vi "Sweep Control Cartesian.vi"() -> ()   [LabVIEW 2019, in "SMO.SweepControl.lvclass"]
doc: "- Priority 0 is the fastest loop\n- You can put multiple scan names in one priority.\n- OFF has to be the last priority\n- Choose an Experiment (Lockin_Sweep, IV, etc) to run at each Scan Setting\n- Open the Exeriment subVIs to choose settings"
uses:
  SMO.SweepControl.lvclass
  Typedefs/Enum - Priority.ctl
  Typedefs/Enum - Action.ctl
  Typedefs/Cluster - ScanControl.ctl
  Typedefs/ScanControl.ctl
  Typedefs/Cluster - ScanParamters.ctl
  Typedefs/ScanParamters.ctl
  Typedefs/Enum - Experiments.ctl
  Typedefs/Sweep Control JSON--Cluster.ctl
  SMO.Control Experiment/SMO.Control Experiment.lvclass
  C:/Program Files (x86)/National Instruments/LabVIEW 2019/user.lib/LevyLab/Instrument Framework/SMOs/Instrument/Instrument.lvclass
  C:/Program Files (x86)/National Instruments/LabVIEW 2019/vi.lib/JKI/JKI SMO/SMO/SMO.lvclass
  Typedefs/Enum - PostAction.ctl
  Typedefs/PostAction.ctl
  Typedefs/Enum - PostAction - 2.ctl
  Typedefs/Cluster - Sweep Control.ctl
panel:
  in  "Scan parameters 2":T1[](array[typedef]) {"Rate" format="%.2f"; "Step" format="%#_6p"; "End" format="%#_6p"; "Start" format="%#_6p"}
  in  "OK":bool
  in  "Experiment Description":string="add your description here"
  in  "Experiment subVI":T5
  in  "Post action (indexing priority)":T6=[enum."Do Nothing", enum."Do Nothing", enum."Do Nothing", enum."Do Nothing"]
  in  "Experiment Folder (## - Description)":string="## - Experiment Folder"
  in  "Scan parameters":T8=[{"Start"=0.0, "End"=0.1, "Step"=0.025, "Rate"=0.0, "Waveform type"=enum."linear", "wait (ms or K)"=250.0, "Address"="Dev2/ao0", "channel"=7}, {"Start"=0.1, "End"=0.2, "Step"=0.025, "Rate"=0.05, "Waveform type"=enum."linear", "wait (ms or K)"=250.0, "Address"="Dev2/ao0", "channel"=2}, {"Start"=0.2, "End"=0.3, "Step"=0.025, "Rate"=2.0, "Waveform type"=enum."linear", "wait (ms or K)"=250.0, "Address"="Dev2/ao0", "channel"=3}, {"Start"=0.0, "End"=10000.0, "Step"=5000.0, "Rate"=0.0, "Waveform type"=enum."linear", "wait (ms or K)"=0.0, "Address"="Dev2/ao0", "channel"=3}] {"Rate" format="%.2f"; "Step" format="%#_6p"; "End" format="%#_6p"; "Start" format="%#_6p"}
  in  "Scan control":T10=[{"Priority"=enum."Priority 0", "Scan name"=enum."Lockin Amplitude"}, {"Priority"=enum."Priority 1", "Scan name"=enum."OFF"}, {"Priority"=enum."Priority 2", "Scan name"=enum."OFF"}, {"Priority"=enum."Priority 3", "Scan name"=enum."OFF"}]
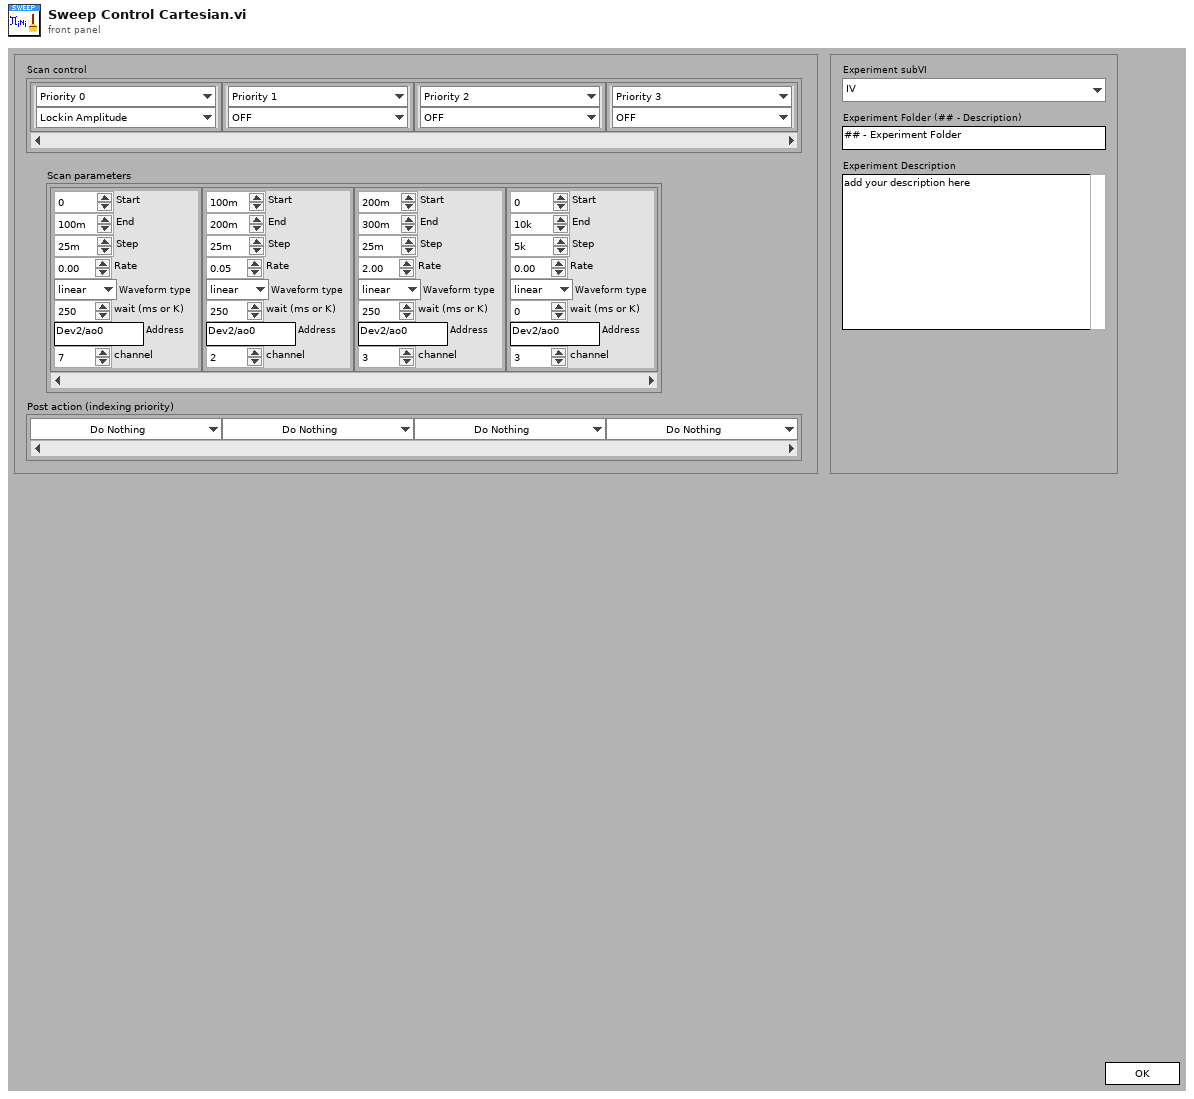
[diagram p1: front panel]
types:
  T1 = typedef "SMO.SweepControl.lvclass/Cluster - Sweep Control.ctl" = cluster{"Start":dbl, "End":dbl, "Step":dbl, "Rate":dbl, "wait (ms/mK)":u32, "Address":string, "Priority":T2, "Scan name":T3, "Post Actions":T4[], "channel":i32}
  T2 = typedef "SMO.SweepControl.lvclass/Enum - Priority.ctl" = enum16{"Priority 0", "Priority 1", "Priority 2", "Priority 3", "Priority 4", "Priority 5"}
  T3 = typedef "SMO.SweepControl.lvclass/Enum - Action.ctl" = enum16{"OFF", "time", "Lockin Amplitude", "Lockin Frequency", "Lockin Bias", "Delay", "Strain", "DAQ Bias", "Magnet Field", "Temperature", "MW f1", "MW f2", "MW Amplitude1", "MW Amplitude2"}
  T4 = typedef "SMO.SweepControl.lvclass/Enum - PostAction - 2.ctl" = enum16{"Do Nothing", "Wait (time)", "Wait (Temperature)", "Wait (<T ; B sweep)", "Wait (Magnet)"}
  T5 = typedef "SMO.SweepControl.lvclass/Enum - Experiments.ctl" = enum16{"IV", "IV_Fast", "THz_DelayLine", "Lockin_Vsg", "Lockin_Sweep", "Lockin_Time", "AI WFM time", "Lockin (experimental)"}
  T6 = typedef "SMO.SweepControl.lvclass/PostAction.ctl" = T7[]
  T7 = typedef "SMO.SweepControl.lvclass/Enum - PostAction.ctl" = enum16{"Do Nothing", "Wait (time)", "Wait (Temperature)", "Wait (<T ; B sweep)", "Wait (Magnet)"}
  T8 = typedef "SMO.SweepControl.lvclass/ScanParamters.ctl" = T9[]
  T9 = typedef "SMO.SweepControl.lvclass/Cluster - ScanParamters.ctl" = cluster{"Start":dbl, "End":dbl, "Step":dbl, "Rate":dbl, "Waveform type":enum16{"linear", "triangle", "power"}, "wait (ms or K)":dbl, "Address":string, "channel":i32}
  T10 = typedef "SMO.SweepControl.lvclass/ScanControl.ctl" = T11[]
  T11 = typedef "SMO.SweepControl.lvclass/Cluster - ScanControl.ctl" = cluster{"Priority":T2, "Scan name":T3}
  T12 = enum32{"Invalid", "Standard", "Closed", "Hidden", "Minimized", "Maximized"}
  T13 = enum32{"invalid app kind", "Development System", "Run Time System", "Student Edition", "Embedded LabVIEW", "Evaluation", "Custom"}
  T14 = cluster{"Core":cluster{"Current VI Reference":refnum<vi>, "Close Panel on Exit?":bool}, "SweepControl":refnum<class "SMO.SweepControl.lvclass">}
  T15 = cluster{"Current VI Reference":refnum<vi>, "Close Panel on Exit?":bool}
  T16 = typedef "SMO.SweepControl.lvclass/Sweep Control JSON--Cluster.ctl" = cluster{"Experiment":T5, "Repeat Experiment":i32, "Scan control":T10, "Scan parameters":T8}
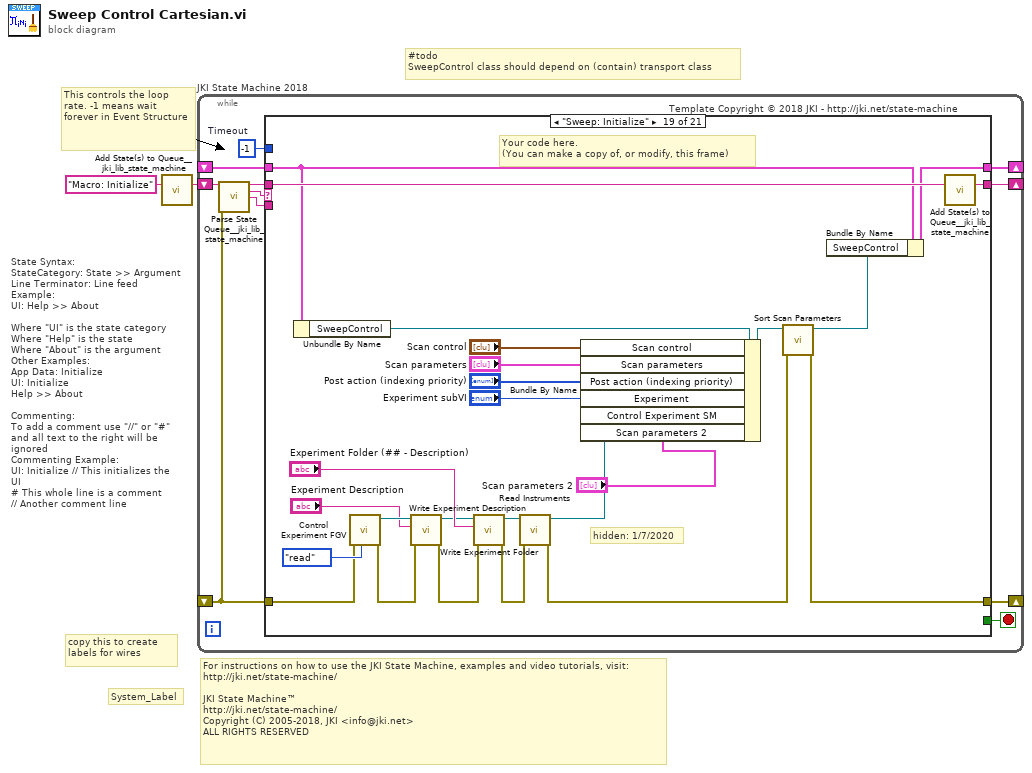
[diagram p0: block diagram]
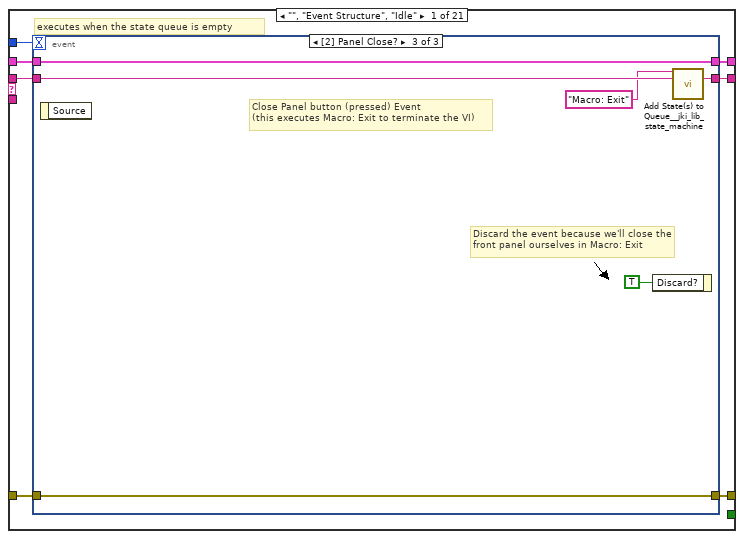
[diagram p2: hidden frame]
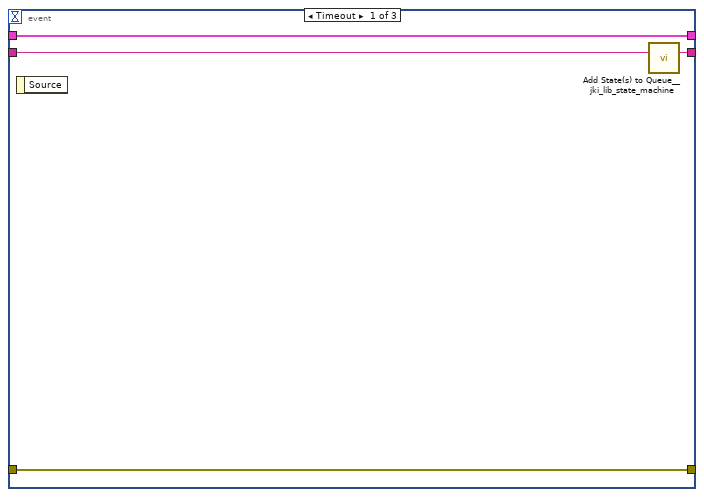
[diagram p3: hidden frame]
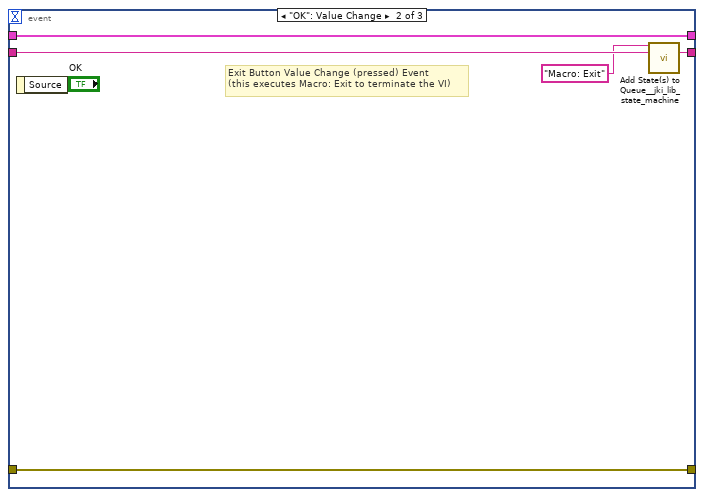
[diagram p4: hidden frame]
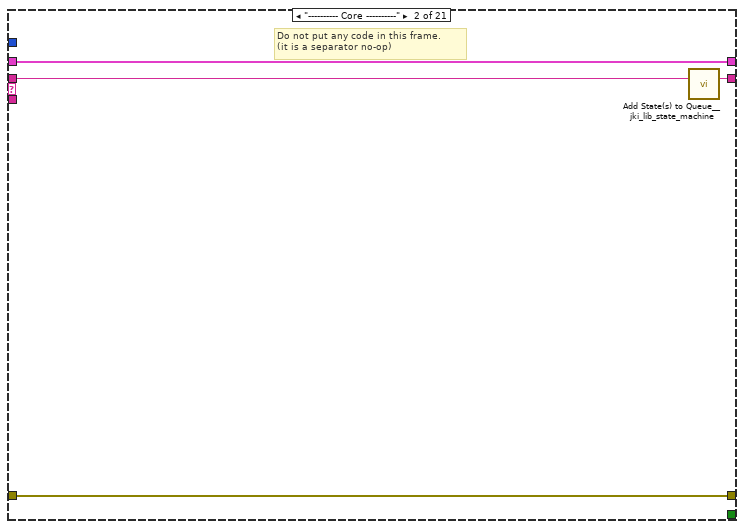
[diagram p5: hidden frame]
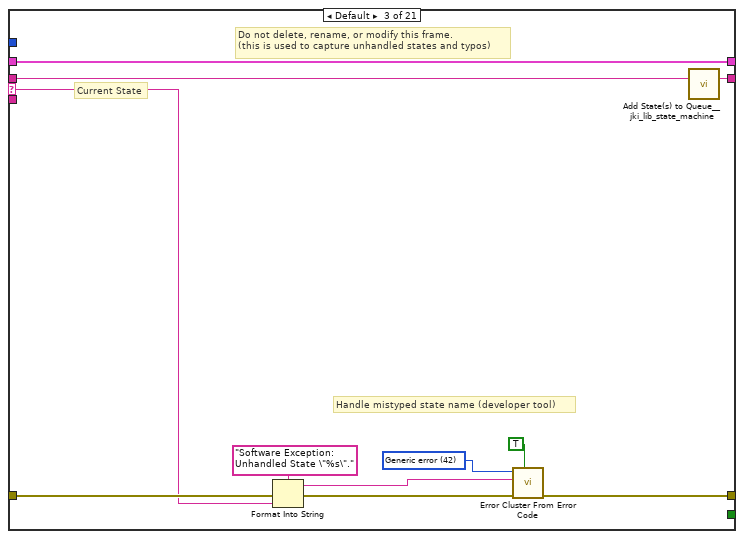
[diagram p6: hidden frame]
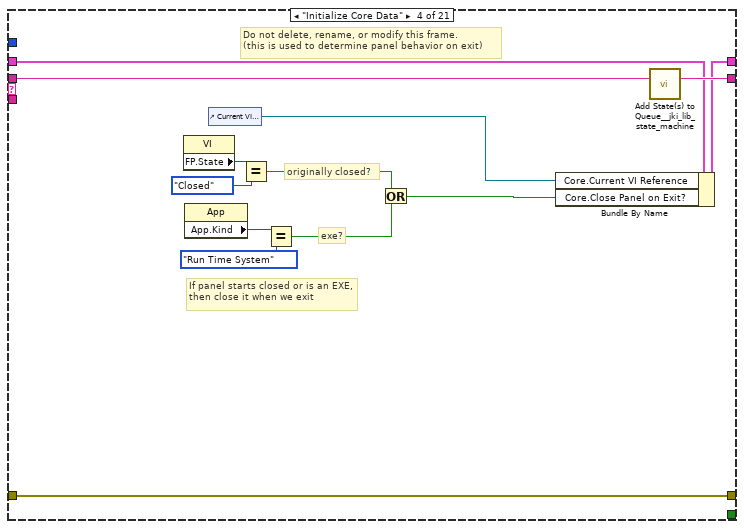
[diagram p7: hidden frame]
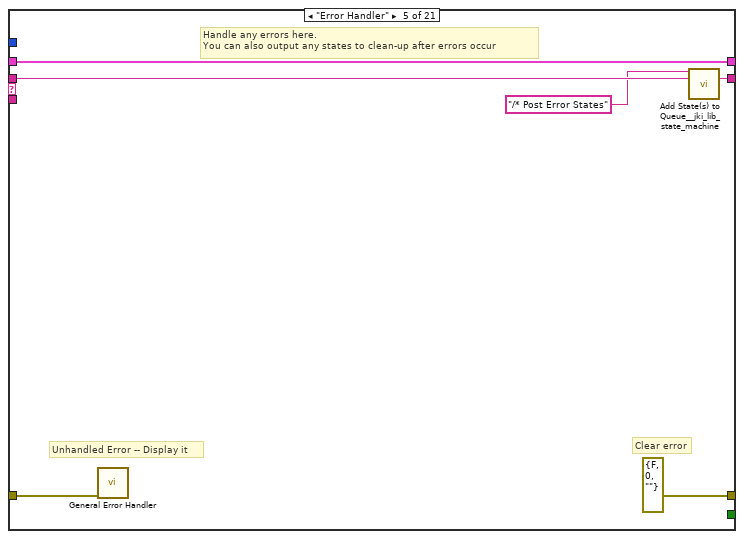
[diagram p8: hidden frame]
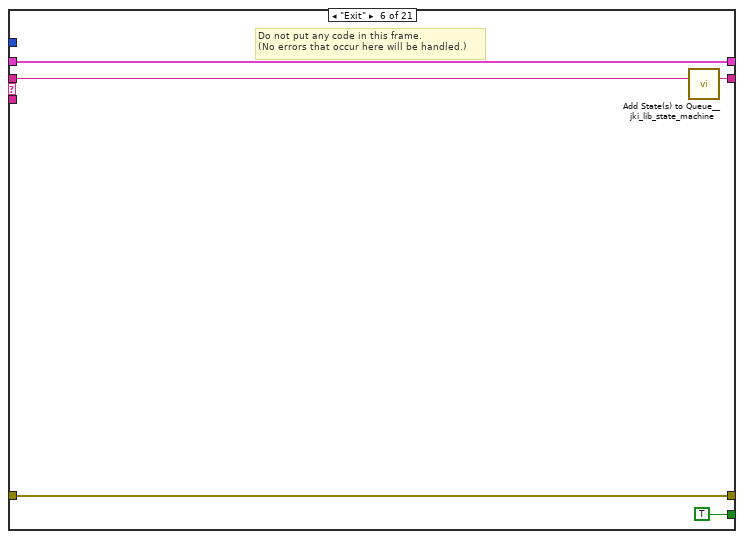
[diagram p9: hidden frame]
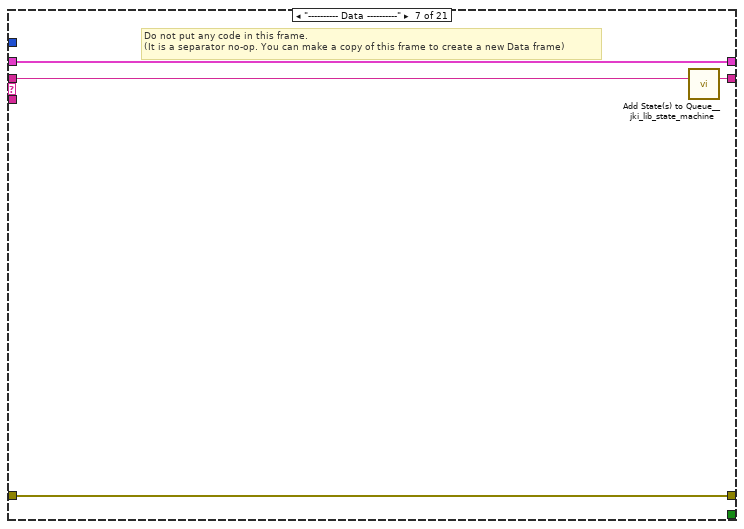
[diagram p10: hidden frame]
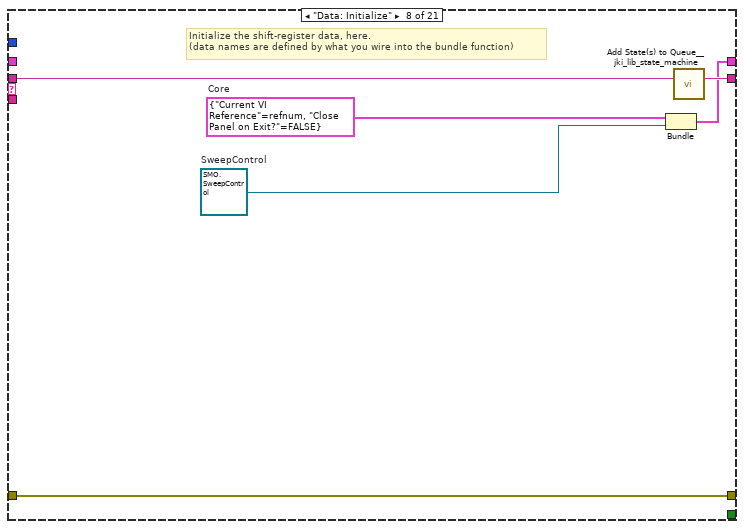
[diagram p11: hidden frame]
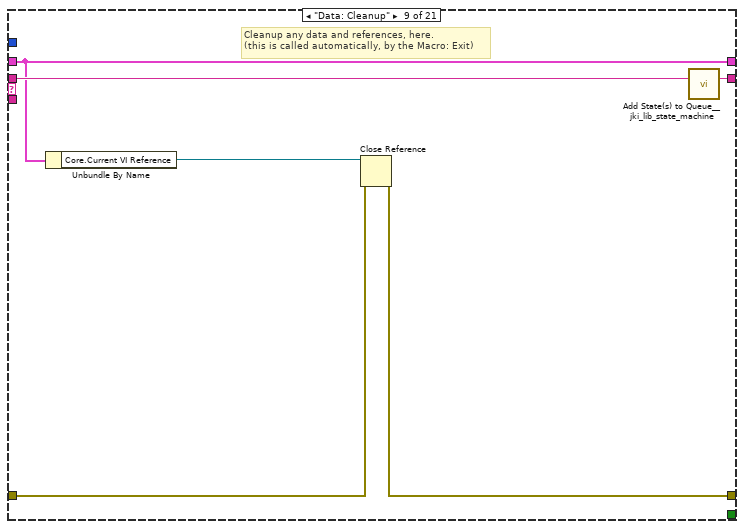
[diagram p12: hidden frame]
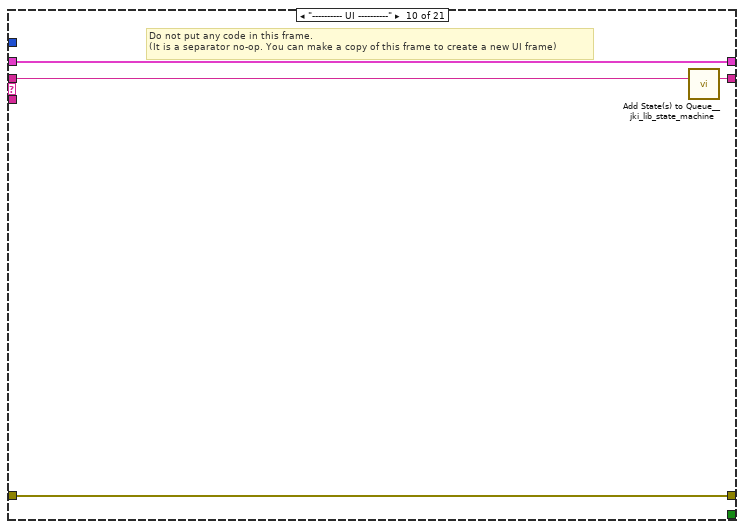
[diagram p13: hidden frame]
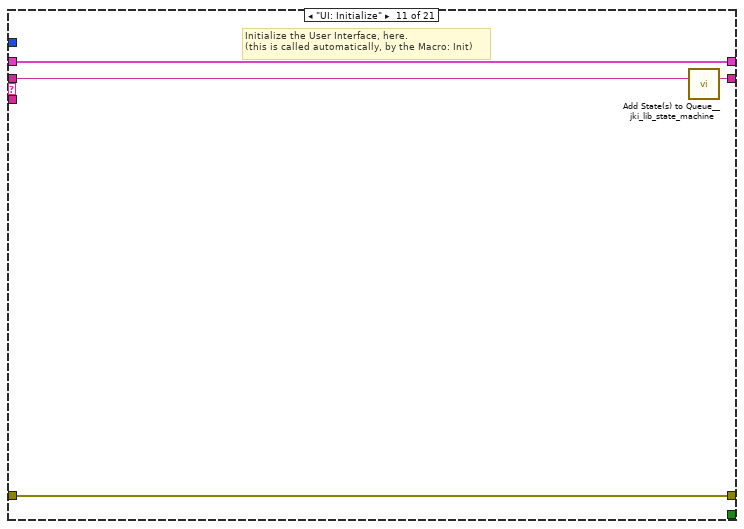
[diagram p14: hidden frame]
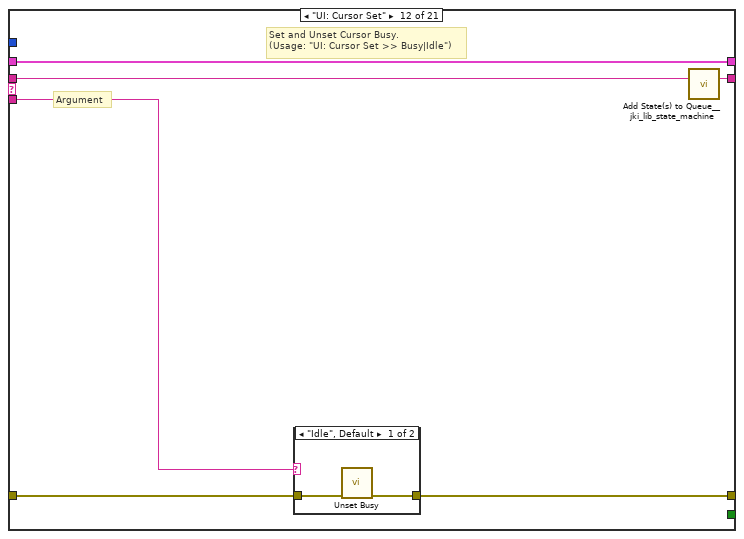
[diagram p15: hidden frame]
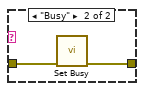
[diagram p16: hidden frame]
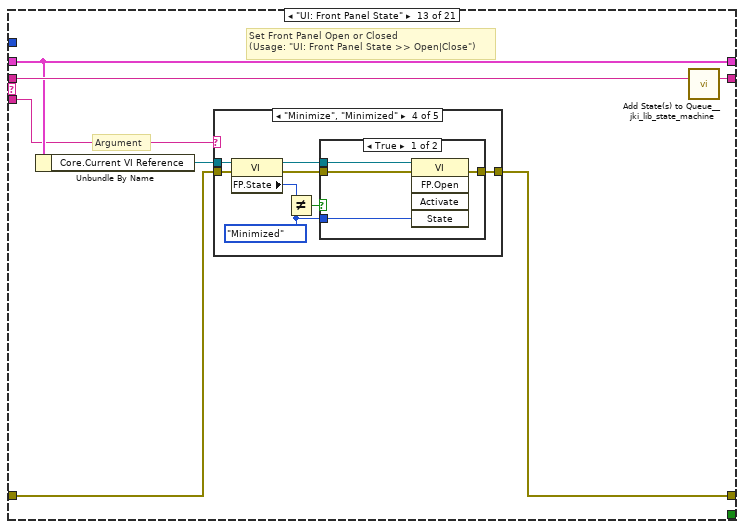
[diagram p17: hidden frame]
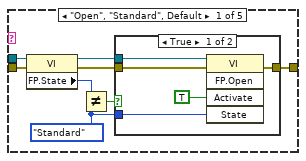
[diagram p18: hidden frame]
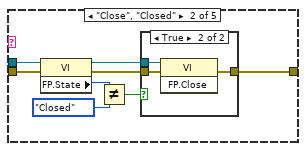
[diagram p20: hidden frame]
diagram:
  # "For instructions on how to use the JKI State Machine, examples and video tutorials, visit:\nhttp://jki.net/state-machine/\n\nJKI State Machine™\nhttp://jki.net/state-machine/\nCopyright (C) 2005-2018, JKI <info@jki.net>\nALL RIGHTS RESERVED"
  # "State Syntax:\nStateCategory: State >> Argument\nLine Terminator: Line feed\nExample:\nUI: Help >> About\n\nWhere \"UI\" is the state category\nWhere \"Help\" is the state\nWhere \"About\" is the argument\nOther Examples:\nApp Data: Initialize\nUI: Initialize\nHelp >> About\n\nCommenting:\nTo add a comment use \"//\" or \"#\" and all text to the right will be ignored\nCommenting Example:\nUI: Initialize // This initializes the UI\n# This whole line is a comment\n// Another comment line"
  # "copy this to create labels for wires"
  # "This controls the loop rate. -1 means wait forever in Event Structure"
  # "System_Label"
  # "#todo\nSweepControl class should depend on (contain) transport class"
  n1 = call <vilib>:"Add State(s) to Queue__jki_lib_state_machine.vi"("State(s) in (\"\")"="Macro: Initialize") -> ("States Out"=w2:string)  [unwired: 14 in]
  n2 = while "JKI State Machine 2018" {
    shift-right: [w6] -> _
    shift-left: _ -> [w5]
    shift-right: [w9] -> _
    shift-left: _ -> [w3]
    shift-right: [w8] -> _
    shift-left: w2 -> [w10]
    stop <- w7 stop-if-true
    w4 = -1  # Timeout
    # "Template Copyright © 2018 JKI - http://jki.net/state-machine"
    n3 = call <vilib>:"Parse State Queue__jki_lib_state_machine.vi"("State Queue"=w10, "Error In (no error)"=w3) -> ("Remaining States"=w12:string, "Current State"=w13:string, "Arguments"=w11:string)  [unwired: 11 in]
    n4 = case shown="\"Sweep: Initialize\"" w13 {
      selector: w13 -> [_ _ w40 _ _ _ _ _ _ _ _ _ _ _ _ _ _ _ _ _ _]
      tunnel: w12 -> [w20 w39 w44 w63 w69 w74 w78 w84 w90 w94 w98 w104 w115 w184 w189 w194 w204 w208 w233 w245 w249]
      tunnel: w11 -> [_ _ _ _ _ _ _ _ _ _ _ w99 w109 _ _ _ _ _ _ _ _]
      tunnel: w5 -> [w18 w36 w42 w56 w66 w72 w75 _ w85 w91 w96 w102 w111 w181 w186 w191 w201 w205 w227 w243 w248]
      tunnel: [w17 w37 w46 w60 errorcluster {"status"=FALSE, "code"=0, "source"=""} ("error out") w71 w76 w81 w86 w92 w95 w100 w112 w182 w187 w192 w202 w206 w225 w238 w247] -> w9
      tunnel: w3 -> [w16 w37 w45 w60 w65 w71 w76 w81 w87 w92 w95 w101 w113 w182 w187 w192 w202 w206 w221 w234 w247]
      tunnel: [w19 w38 w43 w62 w68 w73 w77 w83 w89 w93 w97 w103 w114 w183 w188 w193 w203 w207 w232 w244 w250] -> w8
      tunnel: [_ _ _ _ _ TRUE _ _ _ _ _ _ _ _ _ _ _ _ _ _ _] -> w7
      tunnel: [w15 w36 w42 w61 w66 w72 w75 w82 w85 w91 w96 w102 w111 w181 w186 w191 w201 w205 w226 w243 w248] -> w6
      tunnel: w4 -> [w14 _ _ _ _ _ _ _ _ _ _ _ _ _ _ _ _ _ _ _ _]
      frame "", "Event Structure", "Idle" {
        # "executes when the state queue is empty"
        n5 = event shown="[2] Panel Close?" {
          selector: _ -> [_ _ _]
          dyn-events: _ -> [_ _ _]
          timeout: w14 -> [_ _ _]
          tunnel: w20 -> [w24 w29 w35]
          tunnel: [w23 w28 w34] -> w19
          tunnel: w18 -> [w21 w26 w32]
          tunnel: [w22 w27 w33] -> w17
          tunnel: w16 -> [w22 w27 w33]
          tunnel: [w21 w26 w32] -> w15
          event Timeout {
            n6 = event-data() -> ()  [unwired: 1 in, 1 out]
            n7 = call <vilib>:"Add State(s) to Queue__jki_lib_state_machine.vi"("State(s) in (\"\")"=w24) -> ("States Out"=w23:string)  [unwired: 14 in]
          }
          event "OK": Value Change {
            # "Exit Button Value Change (pressed) Event\n(this executes Macro: Exit to terminate the VI)"
            n8 = event-data() -> ()  [unwired: 1 in, 1 out]
            n9 = call <vilib>:"Add State(s) to Queue__jki_lib_state_machine.vi"("State(s) in Front (\"\")"="Macro: Exit", "State(s) in (\"\")"=w29) -> ("States Out"=w28:string)  [unwired: 13 in]
          }
          event Panel Close? {
            # "Discard the event because we'll close the front panel ourselves in Macro: Exit"
            # "Close Panel button (pressed) Event\n(this executes Macro: Exit to terminate the VI)"
            n10 = event-data() -> ()  [unwired: 1 in, 1 out]
            n11 = event-data("Discard?"=TRUE) -> ()  [unwired: 1 in, 1 out]
            n12 = call <vilib>:"Add State(s) to Queue__jki_lib_state_machine.vi"("State(s) in Front (\"\")"="Macro: Exit", "State(s) in (\"\")"=w35) -> ("States Out"=w34:string)  [unwired: 13 in]
          }
        }
      }
      frame "---------- Core ----------" {
        # "Do not put any code in this frame.\n(it is a separator no-op)"
        n13 = call <vilib>:"Add State(s) to Queue__jki_lib_state_machine.vi"("State(s) in (\"\")"=w39) -> ("States Out"=w38:string)  [unwired: 14 in]
      }
      frame Default {
        w49 = 42 items=["No error", "Argument error", "Memory is full", "Out of zone", "End of file", "File already open", "Generic file I/O error", "File not found", "File permission error", "Disk is full", "Duplicate path", "Too many files open", "System feature not enabled", "Resource file not found", "Cannot add resource", "Resource not found", "Image not found", "Image memory error", "Pen does not exist", "Config type invalid", "Config token not found", "Config parse error", "Config memory error", "Bad external code format", "Bad external code offset", "External code not present", "Null window", "Destroy window error", "Null menu", "Print aborted", "Bad print record", "Print driver error", "Windows error during printing", "Memory error during printing", "Print dialog error", "Generic print error", "Invalid device refnum", "Device not found", "Device parameter error", "Device unit error", "Cannot open device", "Device call aborted", "Generic error", "Cancelled by user", "Object ID too low", "Object ID too high", "Object not in heap", "Unknown heap", "Unknown object (invalid DefProc)", "Unknown object (DefProc not in table)", "Message out of range", "Invalid (null) method", "Unknown message", "Manager call not supported", "Bad address", "Network operation in progress", "Network operation timed out", "Connection is busy", "Network attribute not supported", "Network error", "Address in use", "System out of memory", "Connection aborted", "Connection refused", "Not connected", "Already connected", "Connection closed", "Initialization error (interapplication manager)", "Bad occurrence", "Wait on unbound occurrence handler", "Occurrence queue overflow", "Datalog type conflict", "Unused", "Unrecognized type (interapplication manager)", "Memory corrupt", "Failed to make temporary DLL", "Old CIN version", "Drag socket not found", "Failed to load drop-object", "Failed to register OLE object", "Failed to release OLE object", "Format specifier type mismatch", "Unknown format specifier", "Too few format specifiers", "Too many format specifiers", "Scan failed", "Newer CIN version", "Error converting to variant", "Runtime menu error", "Password tampered", "Variant attribute not found", "Incompatible variant data type", "Event data is not available", "Event Store is not present", "Occurrence is not found", "Event Queue is not created", "Event info is not available", "Refnum passed is NULL", "Error retrieving Class GUID", "Error retrieving CoClass GUID", "Error retrieving TypeLib GUID.", "Bad built application magic bytes.", "Specific driver is different from the specific driver associated with the Logical Name.", "There is no session opened to the class driver.", "Max Error", "MAX - Error with config objects", "MAX - Error loading configuration", "MAX - Group not supported"]
        # "Current State"
        # "Do not delete, rename, or modify this frame.\n(this is used to capture unhandled states and typos)"
        # "Handle mistyped state name (developer tool)"
        n14 = Format Into String(format string="Software Exception: Unhandled State \"%s\"." ("message"), error in=w45, w40) -> (resulting string=w48:string, error out=w47:errorcluster)  [unwired: 1 in]
        n15 = call <vilib>:"Error Cluster From Error Code.vi"("show call chain? (False)"=TRUE, "error in (no error)"=w47, "error message (\"\")"=w48, "error code (0)"=w49) -> ("error out"=w46:errorcluster)  [unwired: 5 in]
        n16 = call <vilib>:"Add State(s) to Queue__jki_lib_state_machine.vi"("State(s) in (\"\")"=w44) -> ("States Out"=w43:string)  [unwired: 14 in]
      }
      frame "Initialize Core Data" {
        # "Do not delete, rename, or modify this frame.\n(this is used to determine panel behavior on exit)"
        # "originally closed?"
        # "exe?"
        # "If panel starts closed or is an EXE, then close it when we exit"
        n17 = property class="VI"() -> ("FP.State"=w53:T12)  [unwired: 2 in, 2 out]
        n18 = property class="App"() -> ("App.Kind"=w59:T13)  [unwired: 2 in, 2 out]
        n19 = control-ref of="Current VI Reference"() -> (w54:refnum<vi>)
        n20 = Equal?(x=w53, y=T12."Closed" ("Front Panel Window:State")) -> (x = y?=w51:bool)
        n21 = Equal?(x=w59, y=T13."Run Time System" ("Application:Kind")) -> (x = y?=w57:bool)
        n22 = Or(x=w51, y=w57) -> (x .or. y?=w55:bool)
        n23 = Bundle By Name(cluster=w56, "Core.Current VI Reference"=w54, "Core.Close Panel on Exit?"=w55) -> (w61:T14)
        n24 = call <vilib>:"Add State(s) to Queue__jki_lib_state_machine.vi"("State(s) in (\"\")"=w63) -> ("States Out"=w62:string)  [unwired: 14 in]
      }
      frame "Error Handler" {
        # "Unhandled Error -- Display it"
        # "Handle any errors here.\nYou can also output any states to clean-up after errors occur"
        # "Clear error"
        n25 = call <vilib>:"General Error Handler.vi"("error in (no error)"=w65) -> ()  [unwired: 10 in, 5 out]
        n26 = call <vilib>:"Add State(s) to Queue__jki_lib_state_machine.vi"("State(s) in Front (\"\")"="/* Post Error States", "State(s) in (\"\")"=w69) -> ("States Out"=w68:string)  [unwired: 13 in]
      }
      frame "Exit" {
        # "Do not put any code in this frame.\n(No errors that occur here will be handled.)"
        n27 = call <vilib>:"Add State(s) to Queue__jki_lib_state_machine.vi"("State(s) in (\"\")"=w74) -> ("States Out"=w73:string)  [unwired: 14 in]
      }
      frame "---------- Data ----------" {
        # "Do not put any code in this frame.\n(It is a separator no-op. You can make a copy of this frame to create a new Data frame)"
        n28 = call <vilib>:"Add State(s) to Queue__jki_lib_state_machine.vi"("State(s) in (\"\")"=w78) -> ("States Out"=w77:string)  [unwired: 14 in]
      }
      frame "Data: Initialize" {
        w79 = refnum<class "SMO.SweepControl.lvclass"> refnum  # SweepControl
        w80 = T15 {"Current VI Reference"=refnum, "Close Panel on Exit?"=FALSE}  # Core
        # "Initialize the shift-register data, here.\n(data names are defined by what you wire into the bundle function)"
        n29 = Bundle("Core"=w80, "SweepControl"=w79) -> (w82:T14)  [unwired: 1 in]
        n30 = call <vilib>:"Add State(s) to Queue__jki_lib_state_machine.vi"("State(s) in (\"\")"=w84) -> ("States Out"=w83:string)  [unwired: 14 in]
      }
      frame "Data: Cleanup" {
        # "Cleanup any data and references, here.\n(this is called automatically, by the Macro: Exit)"
        n31 = Unbundle By Name(w85) -> ("Core.Current VI Reference"=w88:refnum<vi>)
        n32 = Close Reference(reference=w88, error in (no error)=w87) -> (error out=w86:errorcluster)
        n33 = call <vilib>:"Add State(s) to Queue__jki_lib_state_machine.vi"("State(s) in (\"\")"=w90) -> ("States Out"=w89:string)  [unwired: 14 in]
      }
      frame "---------- UI ----------" {
        # "Do not put any code in this frame.\n(It is a separator no-op. You can make a copy of this frame to create a new UI frame)"
        n34 = call <vilib>:"Add State(s) to Queue__jki_lib_state_machine.vi"("State(s) in (\"\")"=w94) -> ("States Out"=w93:string)  [unwired: 14 in]
      }
      frame "UI: Initialize" {
        # "Initialize the User Interface, here.\n(this is called automatically, by the Macro: Init)"
        n35 = call <vilib>:"Add State(s) to Queue__jki_lib_state_machine.vi"("State(s) in (\"\")"=w98) -> ("States Out"=w97:string)  [unwired: 14 in]
      }
      frame "UI: Cursor Set" {
        # "Argument"
        # "Set and Unset Cursor Busy.\n(Usage: \"UI: Cursor Set >> Busy|Idle\")"
        n36 = case shown="\"Idle\", Default" w99 {
          tunnel: w101 -> [w106 w108]
          tunnel: [w105 w107] -> w100
          frame "Idle", Default {
            n37 = call <vilib>:"Unset Busy.vi"("error in (no error)"=w106) -> ("error out"=w105:errorcluster)  [unwired: 10 in]
          }
          frame "Busy" {
            n38 = call <vilib>:"Set Busy.vi"("error in (no error)"=w108) -> ("error out"=w107:errorcluster)  [unwired: 9 in, 1 out]
          }
        }
        n39 = call <vilib>:"Add State(s) to Queue__jki_lib_state_machine.vi"("State(s) in (\"\")"=w104) -> ("States Out"=w103:string)  [unwired: 14 in]
      }
      frame "UI: Front Panel State" {
        # "Argument"
        # "Set Front Panel Open or Closed\n(Usage: \"UI: Front Panel State >> Open|Close\")"
        n40 = Unbundle By Name(w111) -> ("Core.Current VI Reference"=w110:refnum<vi>)
        n41 = case shown="\"Minimize\", \"Minimized\"" w109 {
          tunnel: w113 -> [w121 w136 w147 w160 w173]
          tunnel: [w123 w137 w149 w162 w175] -> w112
          tunnel: w110 -> [w122 w134 w148 w161 w174]
          frame "Open", "Standard", Default {
            w116 = T12."Standard" ("State")
            n42 = property class="VI"(reference=w122, error in=w121) -> (reference out=w119:refnum<vi>, error out=w120:errorcluster, "FP.State"=w118:T12)
            n43 = Not Equal?(x=w118, y=w116) -> (x != y?=w117:bool)
            n44 = case shown="True" w117 {
              tunnel: [w127 w129] -> w123
              tunnel: w120 -> [w126 w129]
              tunnel: w119 -> [w125 _]
              tunnel: w116 -> [w124 _]
              frame True {
                n45 = invoke class="VI" method="FP.Open"(reference=w125, error in=w126, "Activate"=TRUE, "State"=w124) -> (error out=w127:errorcluster)  [unwired: 1 in, 4 out]
              }
              frame False {
              }
            }
          }
          frame "Close", "Closed" {
            n46 = property class="VI"(reference=w134, error in=w136) -> (reference out=w133:refnum<vi>, error out=w135:errorcluster, "FP.State"=w131:T12)
            n47 = Not Equal?(x=w131, y=T12."Closed" ("Front Panel Window:State")) -> (x != y?=w130:bool)
            n48 = case shown="True" w130 {
              tunnel: [w138 w141] -> w137
              tunnel: w135 -> [w138 w140]
              tunnel: w133 -> [_ w139]
              frame False {
              }
              frame True {
                n49 = invoke class="VI" method="FP.Close"(reference=w139, error in=w140) -> (error out=w141:errorcluster)  [unwired: 1 in, 2 out]
              }
            }
          }
          frame "Hidden", "Hide" {
            w142 = T12."Hidden" ("State")
            n50 = property class="VI"(reference=w148, error in=w147) -> (reference out=w145:refnum<vi>, error out=w146:errorcluster, "FP.State"=w144:T12)
            n51 = Not Equal?(x=w144, y=w142) -> (x != y?=w143:bool)
            n52 = case shown="True" w143 {
              tunnel: [w153 w154] -> w149
              tunnel: w146 -> [w152 w154]
              tunnel: w145 -> [w151 _]
              tunnel: w142 -> [w150 _]
              frame True {
                n53 = invoke class="VI" method="FP.Open"(reference=w151, error in=w152, "State"=w150) -> (error out=w153:errorcluster)  [unwired: 2 in, 4 out]
              }
              frame False {
              }
            }
          }
          frame "Minimize", "Minimized" {
            w155 = T12."Minimized" ("State")
            n54 = property class="VI"(reference=w161, error in=w160) -> (reference out=w158:refnum<vi>, error out=w159:errorcluster, "FP.State"=w157:T12)
            n55 = Not Equal?(x=w157, y=w155) -> (x != y?=w156:bool)
            n56 = case shown="True" w156 {
              tunnel: [w166 w167] -> w162
              tunnel: w159 -> [w165 w167]
              tunnel: w158 -> [w164 _]
              tunnel: w155 -> [w163 _]
              frame True {
                n57 = invoke class="VI" method="FP.Open"(reference=w164, error in=w165, "State"=w163) -> (error out=w166:errorcluster)  [unwired: 2 in, 4 out]
              }
              frame False {
              }
            }
          }
          frame "Maximize", "Maximized" {
            w168 = T12."Maximized" ("State")
            n58 = property class="VI"(reference=w174, error in=w173) -> (reference out=w171:refnum<vi>, error out=w172:errorcluster, "FP.State"=w170:T12)
            n59 = Not Equal?(x=w170, y=w168) -> (x != y?=w169:bool)
            n60 = case shown="True" w169 {
              tunnel: [w179 w180] -> w175
              tunnel: w172 -> [w178 w180]
              tunnel: w171 -> [w177 _]
              tunnel: w168 -> [w176 _]
              frame True {
                n61 = invoke class="VI" method="FP.Open"(reference=w177, error in=w178, "State"=w176) -> (error out=w179:errorcluster)  [unwired: 2 in, 4 out]
              }
              frame False {
              }
            }
          }
        }
        n62 = call <vilib>:"Add State(s) to Queue__jki_lib_state_machine.vi"("State(s) in (\"\")"=w115) -> ("States Out"=w114:string)  [unwired: 14 in]
      }
      frame "---------- Macro ----------" {
        # "Do not put any code in this frame.\n(It is a separator no-op. You can make a copy of this frame to create a new Macro frame)"
        n63 = call <vilib>:"Add State(s) to Queue__jki_lib_state_machine.vi"("State(s) in (\"\")"=w184) -> ("States Out"=w183:string)  [unwired: 14 in]
      }
      frame "Macro: Initialize" {
        w185 = "Data: Initialize\nInitialize Core Data\nUI: Initialize\nUI: Front Panel State >> Open\nMacro: Sweep"  # Data: Initialize Initialize Core Data UI: Initialize UI: Front Panel State >> Open Macro: Sweep
        # "Initialization Macro\n(This is called once, when the VI starts)"
        n64 = call <vilib>:"Add State(s) to Queue__jki_lib_state_machine.vi"("State(s) in Front (\"\")"=w185, "State(s) in (\"\")"=w189) -> ("States Out"=w188:string)  [unwired: 13 in]
      }
      frame "Macro: Sweep" {
        # "Do not put any code in this frame.\n(It is a separator no-op. You can make a copy of this frame to create a new Macro frame)"
        n65 = call <vilib>:"Add State(s) to Queue__jki_lib_state_machine.vi"("State(s) in Front (\"\")"="Sweep: Initialize\nSweep: Write JSON File\nSweep: Sweep\nMacro: Exit", "State(s) in (\"\")"=w194) -> ("States Out"=w193:string)  [unwired: 13 in]
      }
      frame "Macro: Exit" {
        # "Exit Macro\n(This is called once, when the VI exits)"
        n66 = Unbundle By Name(w201) -> ("Core.Close Panel on Exit?"=w200:bool)
        n67 = Select(t="UI: Front Panel State >> Close", s=w200, f="") -> (s? t:f=w197:string)
        n68 = call <vilib>:"Add State(s) to Queue__jki_lib_state_machine.vi"("State(s) in (\"\")"=w197, "State(s) at Back (\"\")"="Data: Cleanup\nExit") -> ("States Out"=w195:string)  [unwired: 13 in]
        n69 = call <vilib>:"Add State(s) to Queue__jki_lib_state_machine.vi"("State(s) in Front (\"\")"=w195, "State(s) in (\"\")"=w204) -> ("States Out"=w203:string)  [unwired: 13 in]
      }
      frame "---------- Sweep ----------" {
        # "Template Separator\n(You can make a copy of, or modify, this frame)"
        n70 = call <vilib>:"Add State(s) to Queue__jki_lib_state_machine.vi"("State(s) in (\"\")"=w208) -> ("States Out"=w207:string)  [unwired: 14 in]
      }
      frame "Sweep: Initialize" {
        # "hidden: 1/7/2020"
        # "Your code here.\n(You can make a copy of, or modify, this frame)"
        n71 = Unbundle By Name(w227) -> ("SweepControl"=w224:refnum<class "SMO.SweepControl.lvclass">)
        n72 = call "Control Experiment FGV.vi"("Function"=enum16{"read", "write"}."read", "error in (no error)"=w221) -> ("error out"=w213:errorcluster, "Control Experiment out"=w215:refnum<class "SMO.Control Experiment.lvclass">)  [unwired: 8 in]
        n73 = call "Write Experiment Description.vi"("error in (no error)"=w213, "Experiment Description"="Experiment Description", "Control Experiment"=w215) -> ("error out"=w212:errorcluster, "Control Experiment out"=w211:refnum<class "SMO.Control Experiment.lvclass">)  [unwired: 7 in]
        n74 = call "Write Experiment Folder.vi"("error in (no error)"=w212, "Experiment Folder"="Experiment Folder (## - Description)", "Control Experiment"=w211) -> ("error out"=w217:errorcluster, "Control Experiment out"=w218:refnum<class "SMO.Control Experiment.lvclass">)  [unwired: 7 in]
        n75 = call "Read Instruments.vi"("error in (no error)"=w217, "Control Experiment"=w218) -> ("error out"=w216:errorcluster, "Control Experiment out"=w210:refnum<class "SMO.Control Experiment.lvclass">)  [unwired: 7 in, 1 out]
        n76 = Bundle By Name(cluster=w224, "Scan control"="Scan control", "Scan parameters"="Scan parameters", "Post action (indexing priority)"="Post action (indexing priority)", "Experiment"="Experiment subVI", "Control Experiment SM"=w210, "Scan parameters 2"="Scan parameters 2") -> (w223:refnum<class "SMO.SweepControl.lvclass">)
        n77 = call "Sort Scan Parameters.vi"("error in (no error)"=w216, "SweepControl"=w223) -> ("error out"=w225:errorcluster, "SweepControl"=w219:refnum<class "SMO.SweepControl.lvclass">)  [unwired: 6 in, 2 out]
        n78 = Bundle By Name(cluster=w227, "SweepControl"=w219) -> (w226:T14)
        n79 = call <vilib>:"Add State(s) to Queue__jki_lib_state_machine.vi"("State(s) in (\"\")"=w233) -> ("States Out"=w232:string)  [unwired: 14 in]
      }
      frame "Sweep: Write JSON File" {
        w239 = T16 {"Experiment"=enum."IV", "Repeat Experiment"=0, "Scan control"=[], "Scan parameters"=[]}  # SweepControl
        # "Write JSON File\n(Writes Sweep Control configuration to *.json file)"
        n80 = Unbundle By Name(w243) -> ("SweepControl"=w235:refnum<class "SMO.SweepControl.lvclass">)
        n81 = Unbundle By Name(w235) -> ("Control Experiment SM"=w236)
        n82 = Unbundle By Name(w235) -> ("Scan control"=w242:T10, "Scan parameters"=w241:T8, "Experiment"=w240:T5)
        n83 = Bundle By Name(cluster=w239, "Scan control"=w242, "Scan parameters"=w241, "Experiment"=w240) -> (w237:T16)
        n84 = call "Save JSON File.vi"("error in (no error)"=w234, "Data"=w237, "Control Experiment"=w236) -> ("error out"=w238:errorcluster)  [unwired: 6 in, 2 out]
        n85 = call <vilib>:"Add State(s) to Queue__jki_lib_state_machine.vi"("State(s) in (\"\")"=w245) -> ("States Out"=w244:string)  [unwired: 14 in]
      }
      frame "Sweep: Sweep" {
        # "Your code here.\n(You can make a copy of, or modify, this frame)"
        n86 = Unbundle By Name(w248) -> ("SweepControl"=w246:refnum<class "SMO.SweepControl.lvclass">)
        n87 = call "Sweep Control Loop.vi"("error in (no error)"=w247, "SweepControl in"=w246) -> ()  [unwired: 10 in]
        n88 = call <userlib>:"Cartesian_Experiment.vi"() -> ()  [unwired: 12 in]
        n89 = call <vilib>:"Add State(s) to Queue__jki_lib_state_machine.vi"("State(s) in (\"\")"=w249) -> ("States Out"=w250:string)  [unwired: 14 in]
      }
    }
  }
